vi "COM Stage Test Read.vi"() -> ()   [LabVIEW 2017]
panel:
  out "Position (mm)":dbl
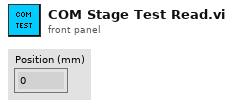
[diagram p1: front panel]
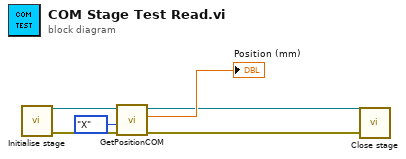
[diagram p0: block diagram]
diagram:
  n1 = call "Initialise stage.vi"() -> ("error out"=w6:errorcluster, "Stage VISA reference"=w5:refnum<visa-resource-name>)  [unwired: 10 in]
  n2 = call "GetPositionCOM.vi"("error in"=w6, "Axis"=enum16{"X", "Y", "Z"}."X", "VISA resource name"=w5) -> ("error out"=w2:errorcluster, "Position (mm)"=→"Position (mm)":dbl, "VISA resource name out"=w1:refnum<visa-resource-name>)  [unwired: 6 in]
  n3 = call "Close stage.vi"("error in"=w2, "VISA resource name"=w1) -> ()  [unwired: 9 in, 1 out]
